vi "Configure List Settings.vi"(6 "List Termination Behavior (1: Last Value)":u16(ring)=1 items=["Original Value", "Last Value"], 7 "List Step Type (1: Auto)":u16(ring)=1 items=["Once", "Auto"], 8 "error in (no error)":errorcluster, 9 "Repeat Continuously (False)":bool, 10 "List Repeat Count (1)":u16=1, 11 "VISA resource name":refnum<visa-resource-name>) -> (0 "error out":errorcluster, 3 "VISA resource name out":refnum<visa-resource-name>)   [LabVIEW 2021, in "Agilent N6900 N7900 Series.lvlib"]
doc: "Configures the commonalities of the list, such as the repetition, step type, and termination behavior."
uses:
  <instrlib>/Agilent N6900 N7900 Series/Agilent N6900 N7900 Series.lvlib
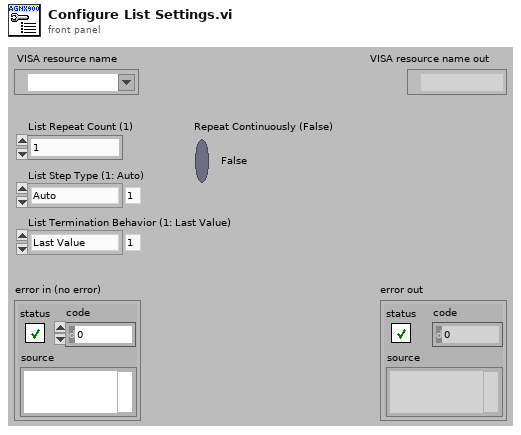
[diagram p1: front panel]
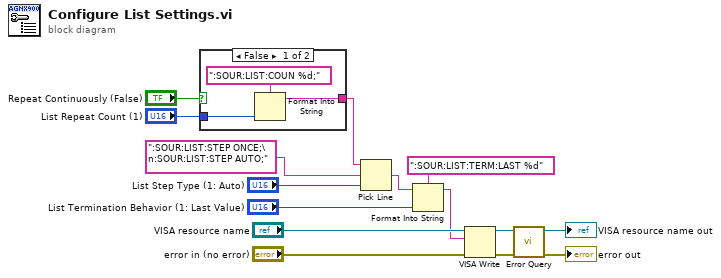
[diagram p0: block diagram]
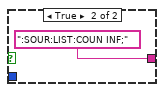
[diagram p2: hidden frame]
diagram:
  n1 = case shown="False" "Repeat Continuously (False)" {
    tunnel: [w16 ":SOUR:LIST:COUN INF;"] -> w1
    tunnel: "List Repeat Count (1)" -> [w18 _]
    frame False {
      n2 = Format Into String(format string=":SOUR:LIST:COUN %d;", w18) -> (resulting string=w16:string)  [unwired: 2 in, 1 out]
    }
    frame True {
    }
  }
  n3 = Pick Line(string ("")=w1, multi-line string=":SOUR:LIST:STEP ONCE;\n:SOUR:LIST:STEP AUTO;", line index="List Step Type (1: Auto)") -> (output string=w4:string)
  n4 = Format Into String(format string=":SOUR:LIST:TERM:LAST %d", initial string=w4, "List Termination Behavior (1: Last Value)") -> (resulting string=w9:string)  [unwired: 1 in, 1 out]
  n5 = VISA Write(VISA resource name="VISA resource name", write buffer=w9, error in (no error)="error in (no error)") -> (VISA resource name out=w12:refnum<visa-resource-name>, error out=w13:errorcluster)  [unwired: 1 out]
  n6 = call <instrlib>:"Error Query.vi"("error in (no error)"=w13, "VISA resource name"=w12) -> ("error out"=→"error out":errorcluster, "VISA resource name out"=→"VISA resource name out":refnum<visa-resource-name>)  [unwired: 6 in, 2 out]
